vi "runTestScenario.vi"(0 "Digital Input Test  in":refnum<class "Set Motor Power Test.lvclass">, 5 "ILC":refnum<class "ILC.lvclass">, 11 "error in (no error)":errorcluster) -> (4 "Digital Input Test out":refnum<class "Set Motor Power Test.lvclass">, 6 "ILC 2":refnum<class "ILC.lvclass">, 8 "TestExecution":T2, 10 "Result":T1, 15 "error out":errorcluster)   [LabVIEW 2015, in "Set Motor Power Test.lvclass"]
uses:
  Set Motor Power Test.lvclass
  Typedefs/TestExecution.ctl
  Typedefs/PassFailTest.ctl
  <userlib>/Common/ILC/ILC/ILC.lvclass
  Typedefs/WriteLogMessageInput.ctl
  Typedefs/TestScenarioTypes.ctl
  Set Motor Power Test.lvclass/Set Motor Power Test.ctl
  Model/TestLog/ITestLog/ITestLog.lvclass
  Model/ConfigureILCStrategy/IConfigureILCStrategy/IConfigureILCStrategy.lvclass
  Typedefs/ILCBTTypedefs.lvlib
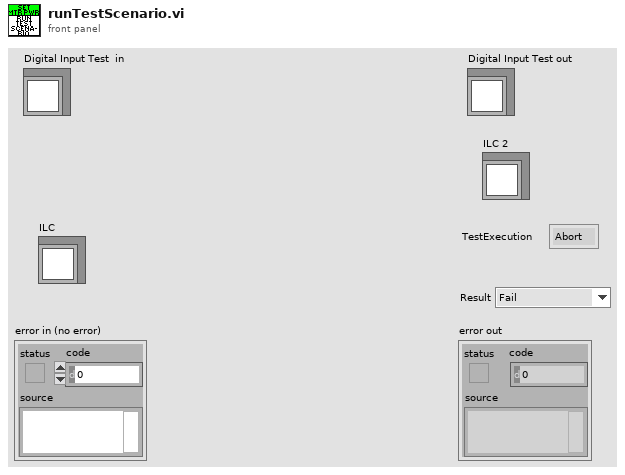
[diagram p1: front panel]
types:
  T1 = typedef "ILCBTTypedefs.lvlib/PassFailTest.ctl" = enum16{"Fail", "Pass", "NA"}
  T2 = typedef "ILCBTTypedefs.lvlib/TestExecution.ctl" = enum16{"Abort", "Continue"}
  T3 = typedef "ILCBTTypedefs.lvlib/WriteLogMessageInput.ctl" = cluster{"Test Scenario":T4, "Description":string, "Actual Value":string, "Data File":string, "Result":T1}
  T4 = typedef "ILCBTTypedefs.lvlib/TestScenarioTypes.ctl" = enum16{"+3.3VD", "+5.1V", "+24V", "RELVALV1", "RELVALV2", "Verify DAC_A = -1.00A", "Verify DAC_A = -0.75A", "Verify DAC_A = -0.50A", "Verify DAC_A = -0.25A", "Verify DAC_A = 0.00A", "Verify DAC_A = 0.25A", "Verify DAC_A = 0.50A", "Verify DAC_A = 0.75A", "Verify DAC_A = 1.00A", "Verify DAC_B = -1.00A", "Verify DAC_B = -0.75A", "Verify DAC_B = -0.50A", "Verify DAC_B = -0.25A", "Verify DAC_B = 0.00A", "Verify DAC_B = 0.25A", "Verify DAC_B = 0.50A", "Verify DAC_B = 0.75A", "Verify DAC_B = 1.00A", "Set DAC_A = -1.00A", "Set DAC_A = -0.75A", "Set DAC_A = -0.50A", "Set DAC_A = -0.25A", "Set DAC_A = 0.00A", "Set DAC_A = 0.25A", "Set DAC_A = 0.50A", "Set DAC_A = 0.75A", "Set DAC_A = 1.00A", "Set DAC_B = -1.00A", "Set DAC_B = -0.75A", "Set DAC_B = -0.50A", "Set DAC_B = -0.25A", "Set DAC_B = 0.00A", "Set DAC_B = 0.25A", "Set DAC_B = 0.50A", "Set DAC_B = 0.75A", "Set DAC_B = 1.00A", "Set MTR_PWR = On", "Set MTR_PWR = Off"}
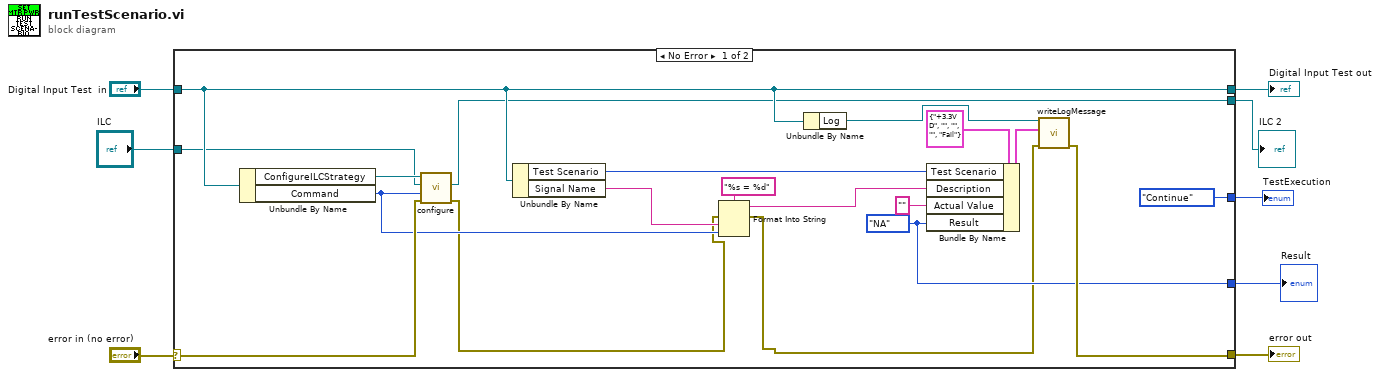
[diagram p0: block diagram]
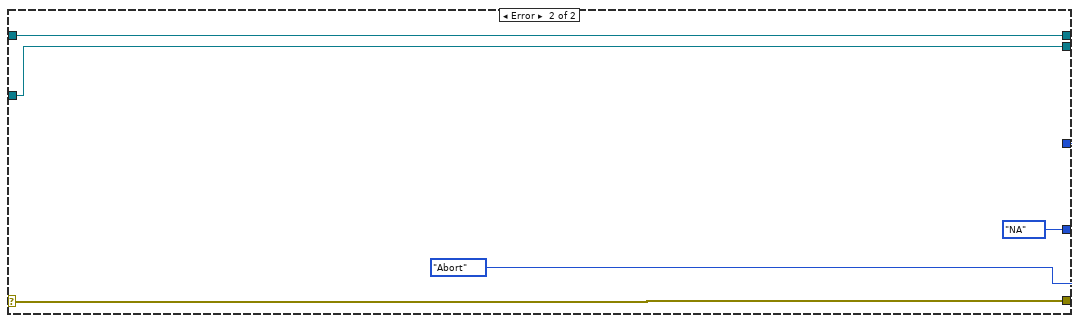
[diagram p2: hidden frame]
diagram:
  n1 = case shown="No Error" "error in (no error)" {
    selector: "error in (no error)" -> [w16 w32]
    tunnel: [w27 w32] -> w7
    tunnel: [TestExecution."Continue" ("TestExecution") TestExecution."Abort" ("TestExecution")] -> w6
    tunnel: "Digital Input Test  in" -> [w18 w30]
    tunnel: [w18 w30] -> w4
    tunnel: "ILC" -> [w15 w29]
    tunnel: [w12 PassFailTest."NA" ("Result")] -> w2
    tunnel: [w10 w29] -> w1
    frame No Error {
      w12 = PassFailTest."NA" ("Result")
      n2 = Unbundle By Name(w18) -> ("ConfigureILCStrategy"=w25:refnum<class "IConfigureILCStrategy.lvclass">, "Command"=w14:u16)
      n3 = call-dynamic "configure.vi"("error in (no error)"=w16, "Value"=w14, "ILC"=w15, "IConfigureILCStrategy in"=w25) -> ("error out"=w11:errorcluster, "ILC 2"=w10:refnum<class "ILC.lvclass">)  [unwired: 5 in, 1 out]
      n4 = Unbundle By Name(w18) -> ("Test Scenario"=w20:T4, "Signal Name"=w24:string)
      n5 = Format Into String(format string="%s = %d", error in=w11, w24, w14) -> (resulting string=w21:string, error out=w9:errorcluster)  [unwired: 1 in]
      n6 = Unbundle By Name(w18) -> ("Log"=w17:refnum<class "ITestLog.lvclass">)
      n7 = Bundle By Name(cluster=T3 {"Test Scenario"=enum."+3.3VD", "Description"="", "Actual Value"="", "Data File"="", "Result"=enum."Fail"} ("WriteLogMessageInput"), "Test Scenario"=w20, "Description"=w21, "Actual Value"="", "Result"=w12) -> (w22:T3)
      n8 = call-dynamic "writeLogMessage.vi"("error in (no error)"=w9, "WriteLogMessageInput"=w22, "ITestLog in"=w17) -> ("error out"=w27:errorcluster)  [unwired: 7 in, 1 out]
    }
    frame Error {
    }
  }
  "Digital Input Test out" <- w4
  "error out" <- w7
  "TestExecution" <- w6
  "Result" <- w2
  "ILC 2" <- w1
